vi "Read Linkage Errors.vi"(8 "error in (no error)":errorcluster, 11 "Test Runner in":refnum<class "Test Runner.lvclass">) -> (0 "error out":errorcluster, 2 "Linkage Errors":errorcluster[](array[cluster]), 3 "Test Runner out":refnum<class "Test Runner.lvclass">)   [LabVIEW 2013, in "Caraya.lvlib" / "Test Runner.lvclass"]
uses:
  Test Runner.lvclass
  Test Runner.lvclass/Test Runner.ctl
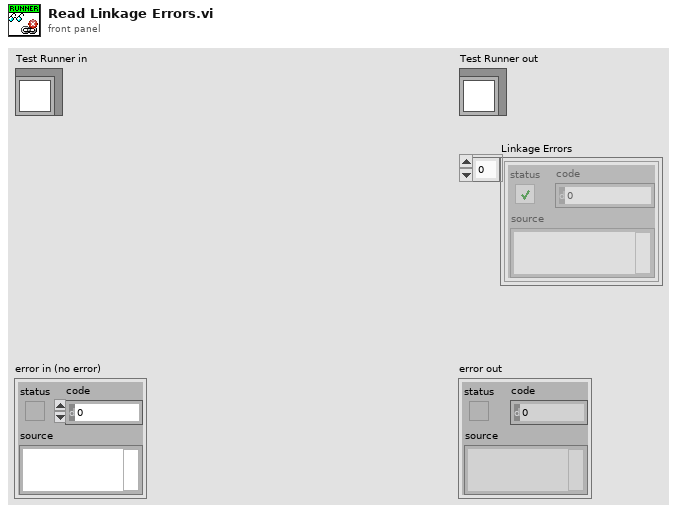
[diagram p1: front panel]
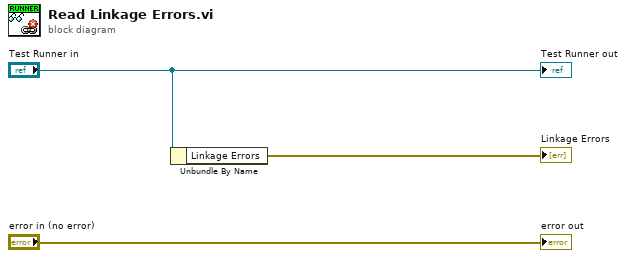
[diagram p0: block diagram]
diagram:
  n1 = Unbundle By Name("Test Runner in") -> ("Linkage Errors"=→"Linkage Errors":errorcluster[])
  "error out" <- "error in (no error)"
  "Test Runner out" <- "Test Runner in"
